vi "Module Interface.vi"(9 "rSubPanel":refnum<vi>, 10 "模块定义":T1={"模块名称"="系统", "项定义"=[{"项名"="设置", "符号图形路径"=path "D:/GitHub/UI-Frame/Pictures/Setting.png"}]}) -> ()   [LabVIEW 2020, in "Grouped Interface.lvlib"]
doc: "This template is based off of the Queued Message Handler design pattern and the Queued Message Handler project template that ships with LabVIEW.\n\nThe main difference is that the queue is private to this module and communication between modules is performed via Broadcast and Request events.\n\nRequest events are wrapped in public API methods and are handled in the Event Handling Loop (EHL) of this VI. Any module can register for Broadcast events sent by this module. The EHL generates messages based on user interface actions.\n\nThe Message Handling Loop (MHL) processes messages generated by the EHL, or by other messages. The messages are string values, so new messages can be added easily to the Message Cases case structure in the MHL. Each message cluster can also provide an optional value for Message Data, which is a variant that can be converted to whatever message-specific data is required.\n_____\nBased on DQMH Project Template 7.0.1.1316."
uses:
  Grouped Interface.lvlib
  <vilib>/Utility/miscctls.llb/LVRectTypeDef.ctl
  Module Definition--cluster.ctl
  Function Item--cluster.ctl
  <vilib>/Utility/miscctls.llb/LVPointTypeDef.ctl
  Window Size Change Arguments--cluster.ctl
  Item Selected Arguments--cluster.ctl
  50509386-df6b-4aff-9ba7-6a02358ed2a7.vi
  9a1344ca-f08d-4af5-a95b-0a8b33b9373c.vi
  7b477b35-5c05-4333-a059-2302209bca0e.vi
  3a33a204-8fa2-46f4-980e-14e97128f476.vi
  233c5268-b16d-435e-a8e5-754348a8c1c8.vi
  191d84f1-7d0a-4105-9754-8d98ffe8b58e.vi
  <userlib>/_NEVSTOP/Communicable State Machine(CSM)/AdvanceAPI/CSM - Revert Arguments-Safe String.vi
  <userlib>/_NEVSTOP/Communicable State Machine(CSM)/_Shared/Trim Single-line Text.vi
  <userlib>/_NEVSTOP/Communicable State Machine(CSM)/AdvanceAPI/CSM - Make String Arguments Safe.vi
  <userlib>/_NEVSTOP/Communicable State Machine(CSM)/AdvanceAPI/CSM - Break Down Multiple States String.vi
  <userlib>/_NEVSTOP/Communicable State Machine(CSM)/AdvanceAPI/CSM - Compact Multiple States.vi
  <userlib>/_NEVSTOP/Communicable State Machine(CSM)/AdvanceAPI/CSM - Keywords.vi
  <userlib>/_NEVSTOP/Communicable State Machine(CSM)/addons/API-String-Arugments-Support/_Support/Data To API String Arguments.vi
  <userlib>/_NEVSTOP/Communicable State Machine(CSM)/addons/API-String-Arugments-Support/_Support/Convert API String Arguments to Data(variant).vi
  <userlib>/_NEVSTOP/Communicable State Machine(CSM)/Communicable State Machine.lvlib
panel:
  out "窗口边界":T3
  in  "界面单元":T4={"ModuleName"="", "FunctionList"=0, "展收按钮"=TRUE, "Spacer"=""}
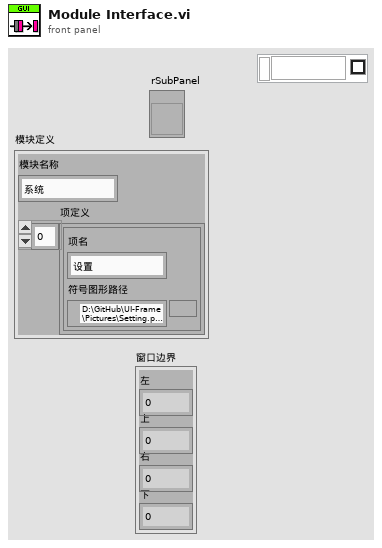
[diagram p1: front panel]
types:
  T1 = typedef "Grouped Interface.lvlib/Module Definition--cluster.ctl" = cluster{"模块名称":string, "项定义":T2[]}
  T2 = typedef "Grouped Interface.lvlib/Function Item--cluster.ctl" = cluster{"项名":string, "符号图形路径":path}
  T3 = typedef "LVRectTypeDef.ctl" = cluster{"Left":i16, "Top":i16, "Right":i16, "Bottom":i16}
  T4 = cluster{"ModuleName":string, "FunctionList":i32, "展收按钮":bool, "Spacer":string}
  T5 = enum32{"Invalid", "Standard", "Closed", "Hidden", "Minimized", "Maximized"}
  T6 = enum32{"invalid app kind", "Development System", "Run Time System", "Student Edition", "Embedded LabVIEW", "Evaluation", "Custom"}
  T7 = typedef "LVPointTypeDef.ctl" = cluster{"Horizontal":i16, "Vertical":i16}
  T8 = typedef "Grouped Interface.lvlib/Window Size Change Arguments--cluster.ctl" = cluster{"Module Name":string, "Window Size":T3}
  T9 = typedef "Grouped Interface.lvlib/Item Selected Arguments--cluster.ctl" = cluster{"Module Name":string, "Item Name":string}
  T10 = cluster{"Item Name":string, "New Item Name":string}
  T11 = typedef "Communicable State Machine.lvlib/_CSM_Response Source Message.ctl" = cluster{"‘State":string, "’Arguments":string, "’Error":errorcluster}
  T12 = cluster{"Current VI Reference":refnum<vi>, "Close Panel on Exit?":bool}
  T13 = cluster{"Core":cluster{"Current VI Reference":refnum<vi>, "Close Panel on Exit?":bool}, "界面单元":refnum<vi>, "ModuleName":refnum<vi>, "FunctionList":refnum<vi>, "Disabled Items":string[]}
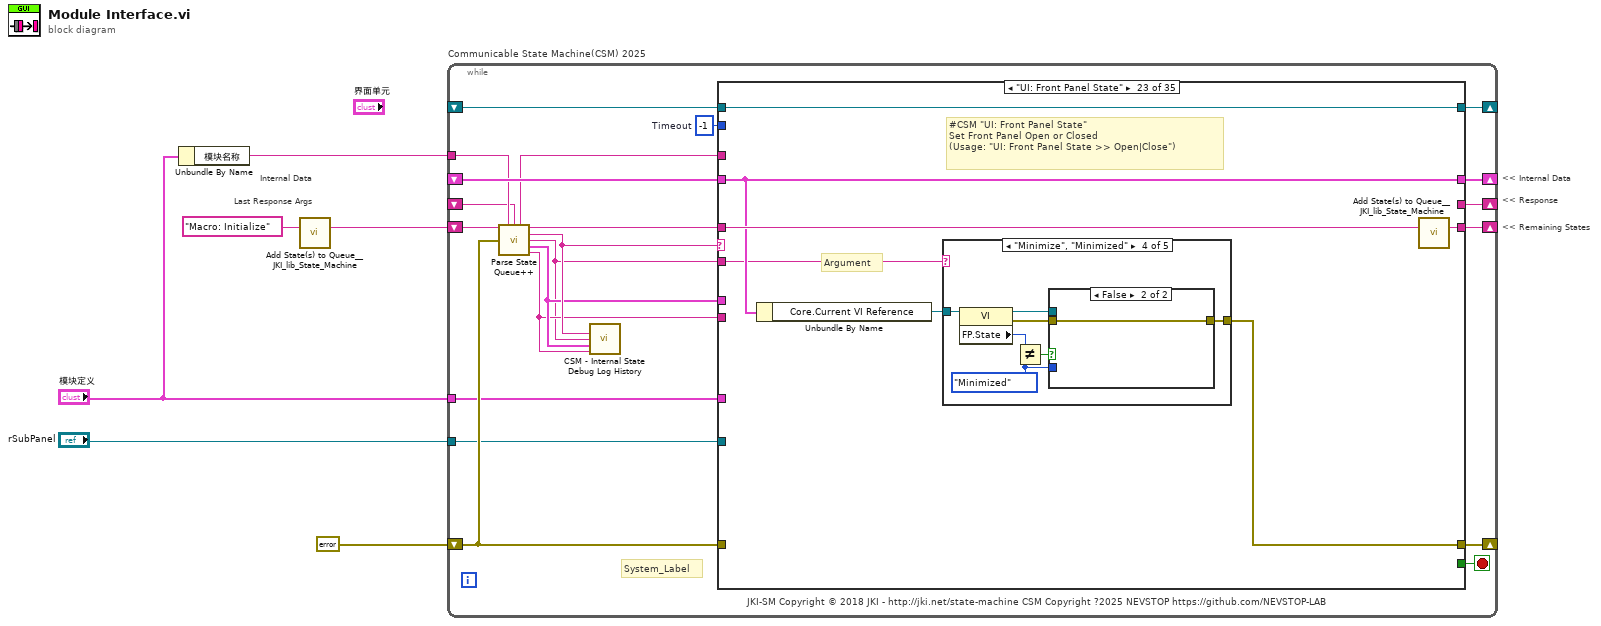
[diagram p0: block diagram]
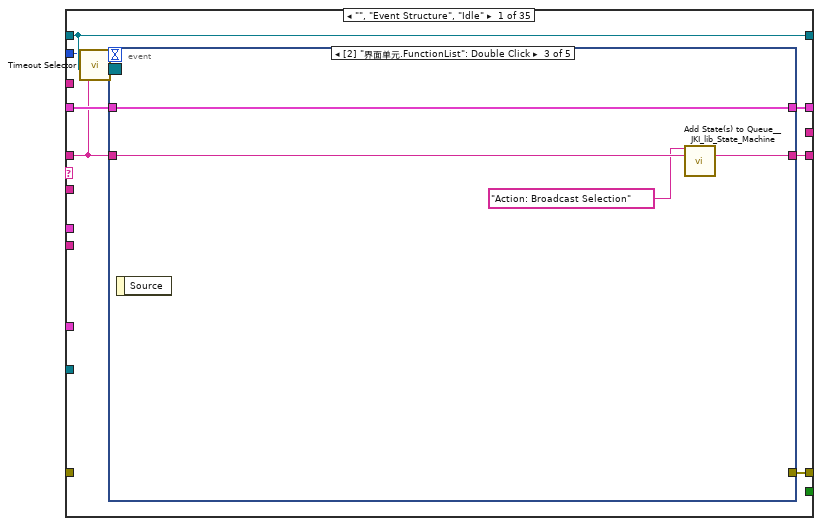
[diagram p2: hidden frame]
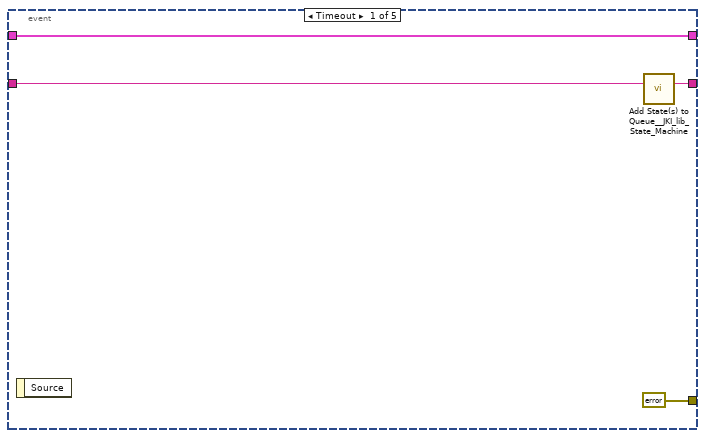
[diagram p3: hidden frame]
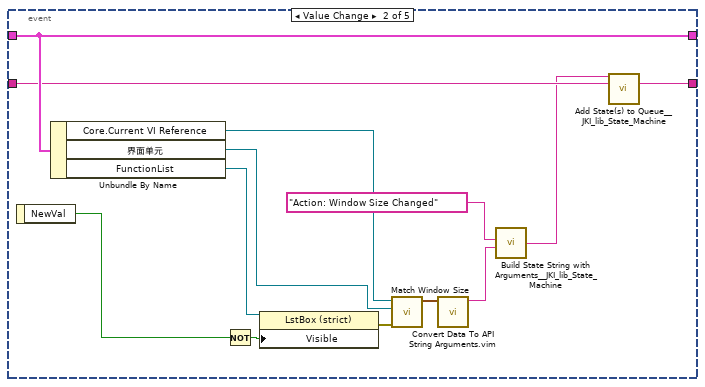
[diagram p4: hidden frame]
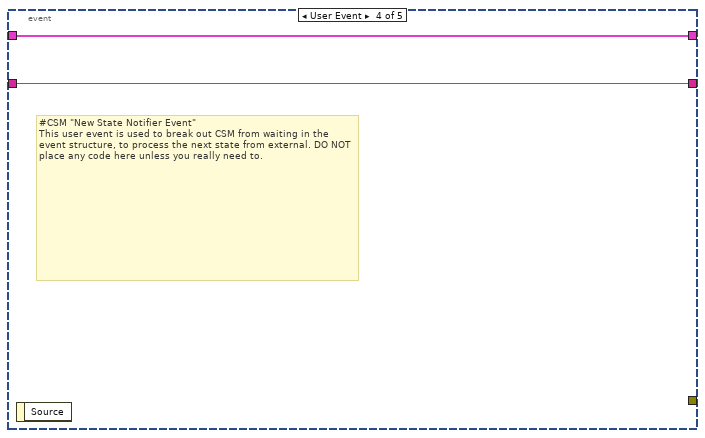
[diagram p5: hidden frame]
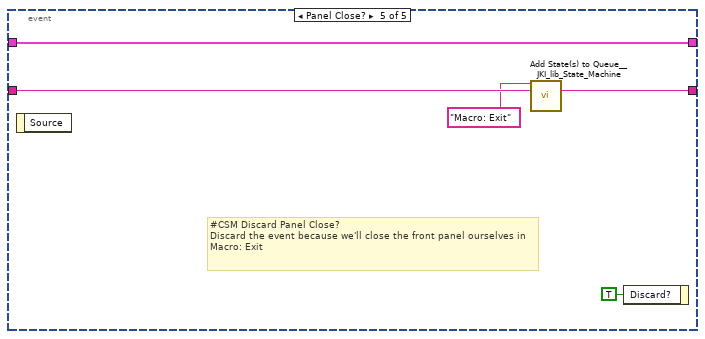
[diagram p6: hidden frame]
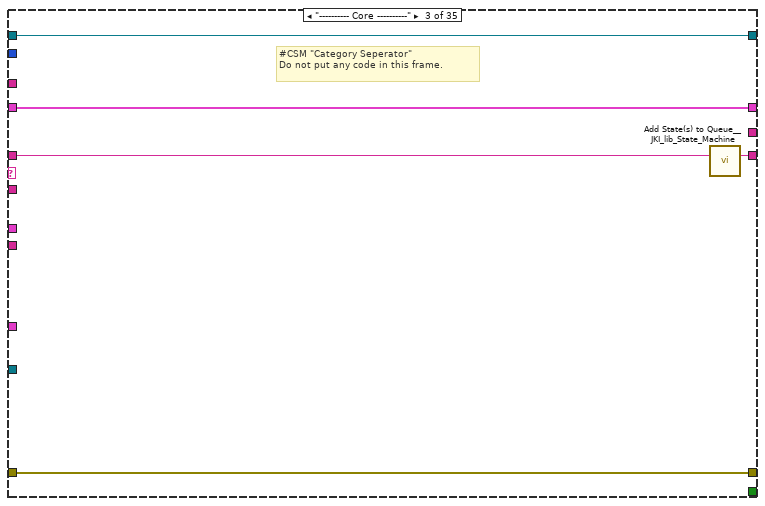
[diagram p8: hidden frame]
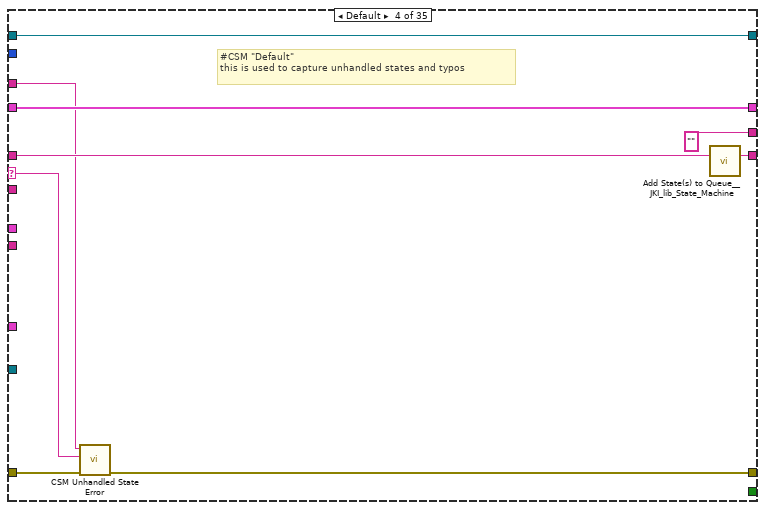
[diagram p9: hidden frame]
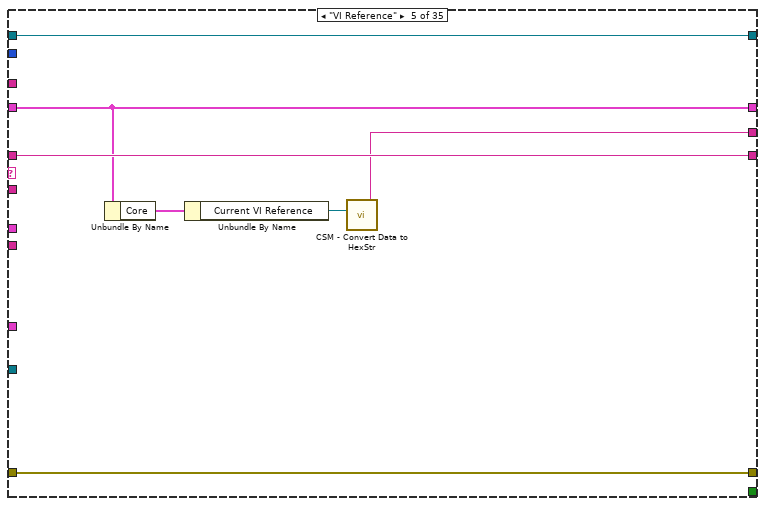
[diagram p10: hidden frame]
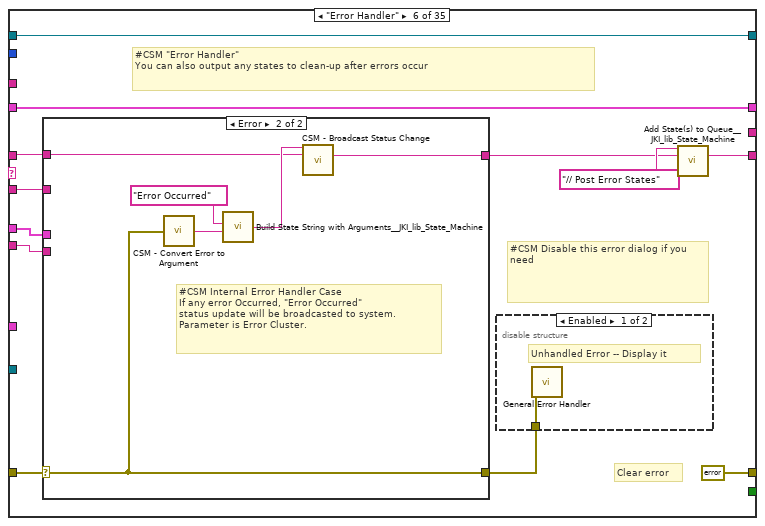
[diagram p11: hidden frame]
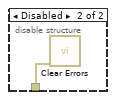
[diagram p12: hidden frame]
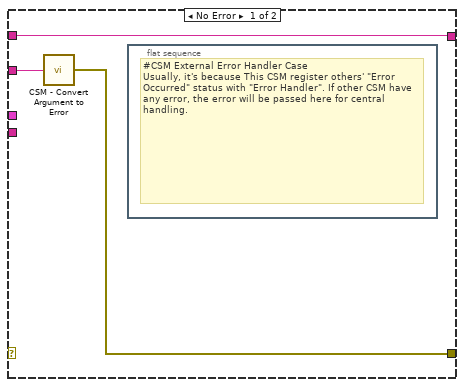
[diagram p13: hidden frame]
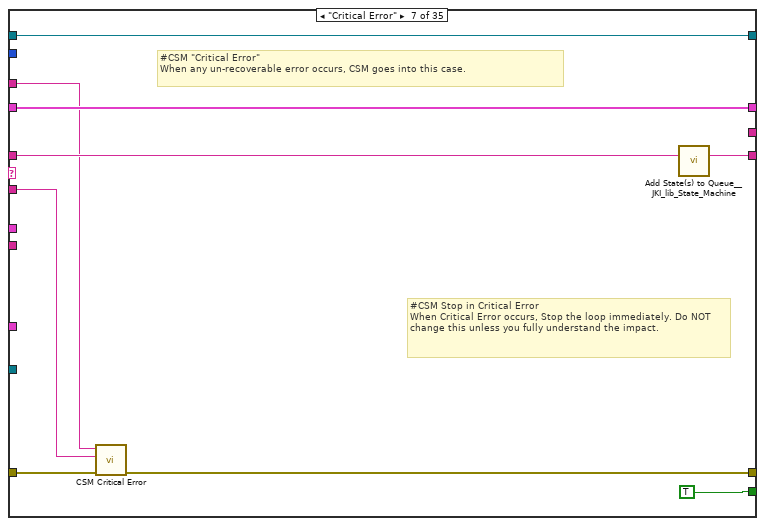
[diagram p14: hidden frame]
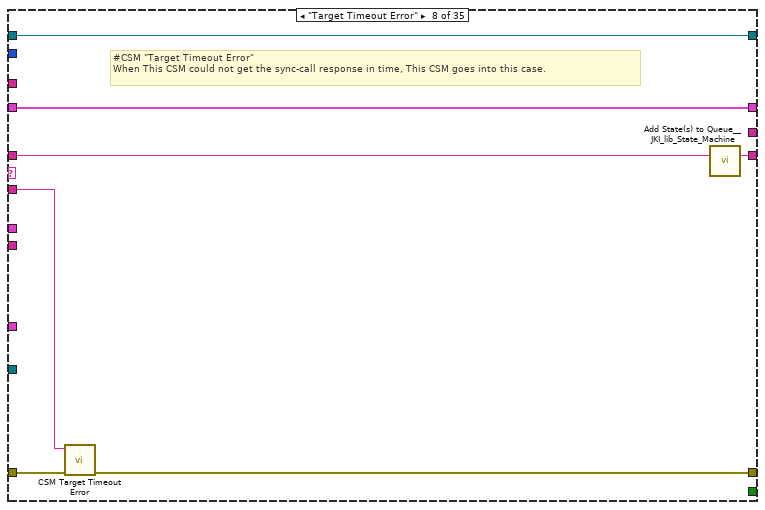
[diagram p15: hidden frame]
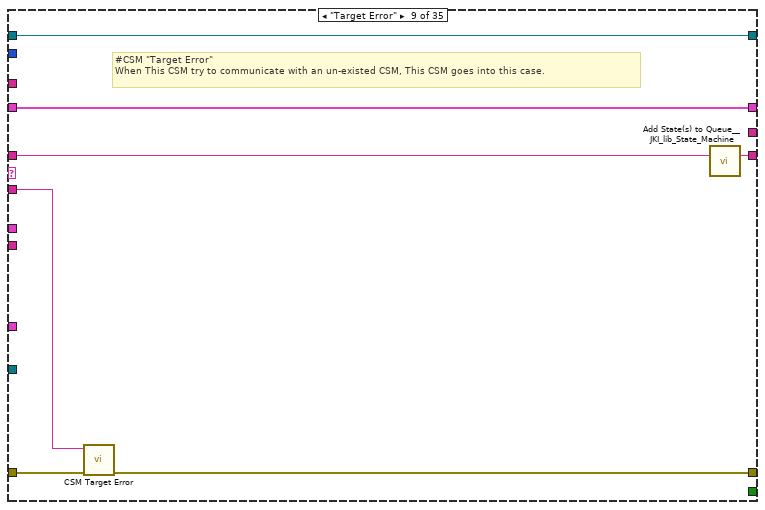
[diagram p16: hidden frame]
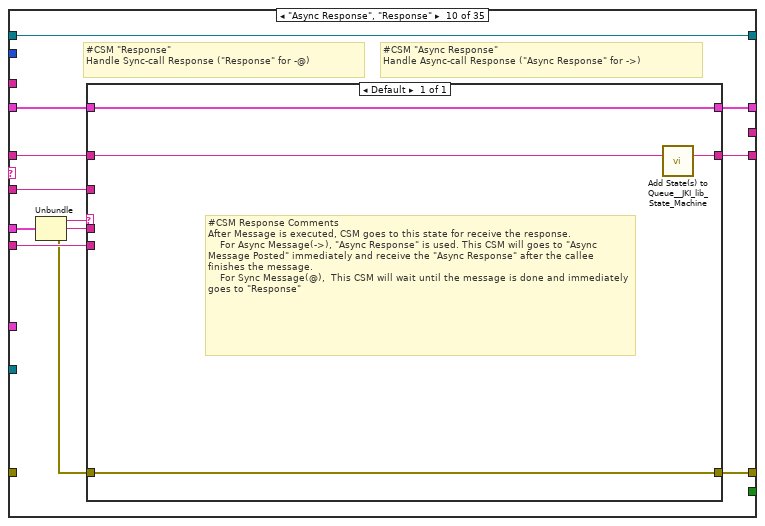
[diagram p17: hidden frame]
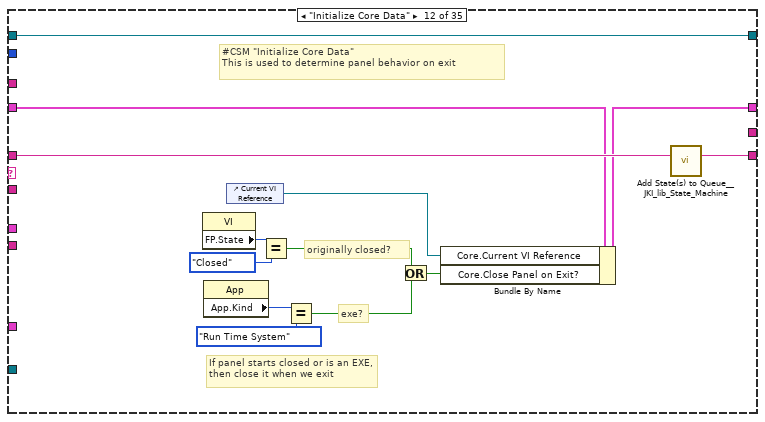
[diagram p19: hidden frame]
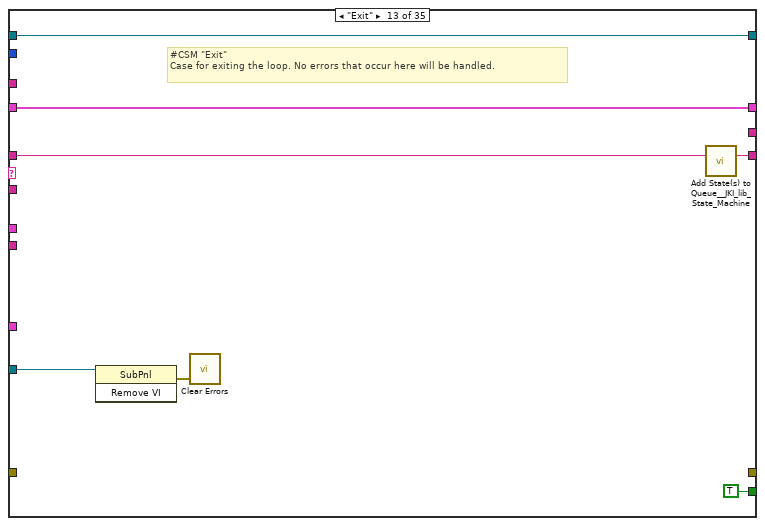
[diagram p20: hidden frame]
diagram:
  # "Last Response Args"
  # "Internal Data"
  # "<< Internal Data"
  # "<< Response"
  # "<< Remaining States"
  n1 = Unbundle By Name("模块定义") -> ("模块名称"=w3:string)
  n2 = call <vilib>:"Add State(s) to Queue__JKI_lib_State_Machine.vi"("State(s) in (\"\")"="Macro: Initialize" ("Init State(\"Macro: Initialize\")")) -> ("States Out"=w4:string)  [unwired: 14 in]
  n3 = while "Communicable State Machine(CSM) 2025" {
    shift-right: [w22] -> _
    shift-left: _ -> [w21]
    shift-right: [w25] -> _
    shift-left: errorcluster {"status"=FALSE, "code"=0, "source"=""} ("error out") -> [w19]
    shift-right: [w24] -> _
    shift-left: w4 -> [w26]
    tunnel: w3 -> [w15]
    shift-right: [w18] -> _
    shift-left: _ -> [w10]
    shift-right: [w17] -> _
    shift-left: _ -> [w16]
    tunnel: "模块定义" -> [w8]
    tunnel: "rSubPanel" -> [w7]
    stop <- w23 stop-if-true
    w20 = -1  # Timeout
    # "System_Label"
    # "JKI-SM Copyright © 2018 JKI - http://jki.net/state-machine CSM Copyright ?2025 NEVSTOP https://github.com/NEVSTOP-LAB"
    n4 = call <userlib>:"Parse State Queue++.vi"("State Queue"=w26, "Name (\"\" to Use UUID)"=w15, "Response Arguments"=w10, "Previous Error"=w19) -> ("Name Used"=w11:string, "Remaining States"=w27:string, "Current State"=w14:string, "Arguments"=w9:string, "Additional Information"=w13:T11, "Source CSM"=w12:string)  [unwired: 6 in]
    n5 = call <userlib>:"CSM - Internal State Debug Log History.vi"("State"=w14, "Arguments (\"\")"=w9, ">> Response Source Message >>"=w13, "Source (\"\")"=w12) -> ()  [unwired: 11 in, 1 out]
    n6 = case shown="\"UI: Front Panel State\"" w14 {
      selector: w14 -> [_ _ _ w74 _ _ _ _ _ _ _ _ _ _ _ _ _ _ _ _ _ _ _ _ _ _ _ _ _ _ _ _ _ _ _]
      tunnel: w27 -> [w28 w66 w71 w80 w86 w92 w118 w126 w133 w143 w152 w165 w172 w176 w185 w191 w195 w202 w206 w210 w230 w236 w247 w311 w316 w327 w330 w334 w337 w341 w352 w356 w389 w409 w432]
      tunnel: w9 -> [_ _ _ _ _ w90 w114 w121 w129 w137 _ _ _ _ _ _ _ _ _ _ _ w232 w242 _ _ _ _ _ _ _ w344 _ w379 w399 w426]
      tunnel: w21 -> [w34 w65 w68 w78 w85 w98 w119 w124 w131 w141 w151 w159 w170 w174 _ w187 w193 w201 w205 w208 w226 w234 w244 w309 w314 w325 w329 w333 w336 w339 w354 w359 w380 w398 w421]
      tunnel: [w33 _ w69 w72 w87 errorcluster {"status"=FALSE, "code"=0, "source"=""} ("error out") w111 w120 w127 w140 _ _ _ _ _ w188 _ w196 w204 _ _ w233 w245 _ _ _ _ _ _ _ _ _ _ _ _] -> w25
      tunnel: w19 -> [_ _ w69 w73 w87 w96 w112 w122 w128 _ _ _ _ _ _ _ _ _ _ _ _ _ _ _ _ _ _ _ _ _ _ _ _ _ _]
      tunnel: [w35 w66 w70 w79 w86 w94 w117 w125 w132 w144 w152 w164 w171 w175 w184 w190 w194 w202 w206 w209 w229 w235 w246 w310 w315 w326 w330 w334 w337 w340 w351 w357 w388 w408 w431] -> w24
      tunnel: [_ _ _ _ _ _ TRUE _ _ _ _ _ TRUE _ _ _ _ _ _ _ _ _ _ _ _ _ _ _ _ _ _ _ _ _ _] -> w23
      tunnel: [w32 w65 w68 w78 w85 w98 w119 w124 w131 w142 w151 w163 w170 w174 w183 w187 w193 w201 w205 w208 w226 w234 w244 w309 w314 w325 w329 w333 w336 w339 w354 w359 w377 w397 w421] -> w22
      tunnel: w20 -> [w30 _ _ _ _ _ _ _ _ _ _ _ _ _ _ _ _ _ _ _ _ _ _ _ _ _ _ _ _ _ _ _ _ _ _]
      tunnel: w12 -> [_ _ _ _ _ w89 _ _ _ w138 _ _ _ _ _ _ _ _ _ _ _ _ _ _ _ _ _ _ _ _ _ _ _ _ _]
      tunnel: w13 -> [_ _ _ _ _ w88 _ _ _ w139 _ _ _ _ _ _ _ _ _ _ _ _ _ _ _ _ _ _ _ _ _ _ _ _ _]
      tunnel: [_ _ _ "" w81 _ _ _ _ _ _ _ _ _ _ _ _ _ _ _ _ _ _ _ _ _ _ "API1 Response" _ _ _ _ _ _ _] -> w18
      tunnel: [w31 w64 w67 w76 w84 w97 w115 w123 w130 w145 w150 w153 w168 w173 w181 w186 w192 w200 w203 w207 w228 w231 w241 w308 w312 w318 w328 w332 w335 w338 w353 w366 w387 w407 w430] -> w17
      tunnel: w16 -> [w31 w64 w67 w76 w84 w97 w115 w123 w130 w145 w150 w153 w168 w173 w181 w186 w192 _ w203 w207 w228 w231 w241 w308 w312 w318 w328 w332 w335 w338 w353 w366 w387 w407 w430]
      tunnel: w11 -> [_ _ _ w75 _ _ w113 _ _ _ _ _ _ _ _ _ _ w199 _ _ _ _ _ _ _ _ _ _ _ _ w347 w355 _ _ _]
      tunnel: w8 -> [_ _ _ _ _ _ _ _ _ _ _ _ _ _ _ _ _ _ _ _ w227 _ _ _ _ _ _ _ _ _ _ _ _ _ _]
      tunnel: w7 -> [_ _ _ _ _ _ _ _ _ _ _ _ w166 _ _ _ _ _ _ _ w221 _ _ _ _ _ _ _ _ _ _ _ _ _ _]
      frame "", "Event Structure", "Idle" {
        n7 = call <userlib>:"Timeout Selector.vi"("Remaining States"=w28, "Timeout Expected"=w30) -> ("Timeout"=w29:i32)  [unwired: 5 in]
        n8 = event shown="[2] \"界面单元.FunctionList\": Double Click" {
          selector: w31 -> [_ _ _ _ _]
          dyn-events: _ -> [_ _ _ _ _]
          timeout: w29 -> [_ _ _ _ _]
          tunnel: w28 -> [w39 w41 w54 w57 w63]
          tunnel: [w38 w42 w55 w57 w62] -> w35
          tunnel: w34 -> [w37 w48 w56 w58 w61]
          tunnel: [errorcluster {"status"=FALSE, "code"=0, "source"=""} ("error out") _ _ _ _] -> w33
          tunnel: [w37 w48 w56 w58 w61] -> w32
          event Timeout {
            n9 = event-data() -> ()  [unwired: 1 in, 1 out]
            n10 = call <vilib>:"Add State(s) to Queue__JKI_lib_State_Machine.vi"("State(s) in (\"\")"=w39) -> ("States Out"=w38:string)  [unwired: 14 in]
          }
          event "界面单元.展收按钮": Value Change {
            n11 = event-data() -> ("NewVal"=w49:bool)  [unwired: 1 in]
            n12 = Unbundle By Name(w48) -> ("Core.Current VI Reference"=w45:refnum<vi>, "界面单元"=w46:refnum<vi>, "FunctionList"=w47:refnum<vi>)
            n13 = Not(x=w49) -> (.not. x?=w51:bool)
            n14 = property class="LstBox (strict)"(reference=w47, "Visible"=w51) -> (error out=w52:errorcluster)  [unwired: 1 in, 1 out]
            n15 = call "Match Window Size.vi"("错误输入（无错误）"=w52, "界面单元"=w46, "VI输入"=w45) -> ("窗口边界"=w50:T3)  [unwired: 7 in, 1 out]
            n16 = call "Convert Data To API String Arguments.vim"("Data"=w50) -> ("API String"=w43:string)  [unwired: 7 in, 1 out]
            n17 = call <vilib>:"Build State String with Arguments__JKI_lib_State_Machine.vi"("Arguments (\"\")"=w43, "State"="Action: Window Size Changed") -> ("State with Arguments"=w40:string)  [unwired: 4 in]
            n18 = call <vilib>:"Add State(s) to Queue__JKI_lib_State_Machine.vi"("State(s) in Front (\"\")"=w40, "State(s) in (\"\")"=w41) -> ("States Out"=w42:string)  [unwired: 13 in]
          }
          event "界面单元.FunctionList": Double Click {
            n19 = event-data() -> ()  [unwired: 1 in, 1 out]
            n20 = call <vilib>:"Add State(s) to Queue__JKI_lib_State_Machine.vi"("State(s) in Front (\"\")"="Action: Broadcast Selection" ("State(s) in Front (\"\")"), "State(s) in (\"\")"=w54) -> ("States Out"=w55:string)  [unwired: 13 in]
          }
          event User Event {
            # "#CSM \"New State Notifier Event\"\nThis user event is used to break out CSM from waiting in the event structure, to process the next state from external. DO NOT place any code here unless you really need to."
            n21 = event-data() -> ()  [unwired: 1 in, 1 out]
          }
          event Panel Close? {
            # "#CSM Discard Panel Close?\nDiscard the event because we'll close the front panel ourselves in Macro: Exit"
            n22 = event-data() -> ()  [unwired: 1 in, 1 out]
            n23 = call <vilib>:"Add State(s) to Queue__JKI_lib_State_Machine.vi"("State(s) in Front (\"\")"="Macro: Exit", "State(s) in (\"\")"=w63) -> ("States Out"=w62:string)  [unwired: 13 in]
            n24 = event-data("Discard?"=TRUE) -> ()  [unwired: 1 in, 1 out]
          }
        }
      }
      frame "CSM Documentation" {
        # "#CSM State Syntax\n\n// Comment line, all text to the right of “//” will be ignored\n// Local Message Example\nDoSth: DoA >> Arguments\n\n// Sync Call Example\nAPI: xxxx >> Arguments -@ TargetModule\n\n// Async Call Example\nAPI: xxxx >> Arguments -> TargetModule\n\n// Async Call without Reply Example\nAPI: xxxx >> Arguments ->| TargetModule\n\n// Broadcast normal status:\nStatus >> StatusArguments  -><status>\n\n// Broadcast Interrupt status:\nInterrupt >> StatusArguments  -><interrupt>\n\n// Register Source Module's status to Handler Module\nStatus@Source Module >> Handler Module@Handler Module -><register>\n\n// Unegister Source Module's status\nStatus@Source Module >> Handler Module -><unregister>"
        # "#CSM README FIRST\n\nCommunicable State Machine(CSM) is a LabVIEW application framework that builds upon JKI State Machine(JKISM). It follows the pattern of JKISM and extends the keywords to describe message communication between modules, including concepts such as Sync-Message, Async-Message, Subscription/Unsubscription of status - essential elements for creating reusable code modules. For more information, please visit the CSM wiki: https://nevstop-lab.github.io/CSM-Wiki/\n\nFor instructions on JKI State Machine, visit: \n    http://jki.net/state-machine/\nFor information about CSM, visit: \n    https://github.com/NEVSTOP-LAB"
        # "#CSM \"Documentation\"\nCase for holding CSM Documenation"
      }
      frame "---------- Core ----------" {
        # "#CSM \"Category Seperator\"\nDo not put any code in this frame."
        n25 = call <vilib>:"Add State(s) to Queue__JKI_lib_State_Machine.vi"("State(s) in (\"\")"=w71) -> ("States Out"=w70:string)  [unwired: 14 in]
      }
      frame Default {
        # "#CSM \"Default\"\nthis is used to capture unhandled states and typos"
        n26 = call <userlib>:"CSM Unhandled State Error.vi"("error in (no error)"=w73, "Undefined State"=w74, "CSM Name"=w75) -> ("error out"=w72:errorcluster)  [unwired: 8 in]
        n27 = call <vilib>:"Add State(s) to Queue__JKI_lib_State_Machine.vi"("State(s) in (\"\")"=w80) -> ("States Out"=w79:string)  [unwired: 14 in]
      }
      frame "VI Reference" {
        n28 = Unbundle By Name(w85) -> ("Core"=w83:T12)
        n29 = Unbundle By Name(w83) -> ("Current VI Reference"=w82:refnum<vi>)
        n30 = call <userlib>:"CSM - Convert Data to HexStr.vi"("Variant"=w82) -> ("HEX String (0-9,A-F)"=w81:string)  [unwired: 8 in]
      }
      frame "Error Handler" {
        # "#CSM Disable this error dialog if you need"
        # "#CSM \"Error Handler\"\nYou can also output any states to clean-up after errors occur"
        # "Clear error"
        n31 = case shown="Error" w96 {
          selector: w96 -> [_ w105]
          tunnel: [w103 w107] -> w93
          tunnel: w92 -> [w103 w106]
          tunnel: [w102 w105] -> w91
          tunnel: w90 -> [w104 _]
          tunnel: w89 -> [_ _]
          tunnel: w88 -> [_ _]
          frame No Error {
            n32 = call <userlib>:"CSM - Convert Argument to Error.vi"("Argument"=w104) -> ("Error"=w102:errorcluster)  [unwired: 4 in]
            n33 = flat-sequence {
              frame #0 {
                # "#CSM External Error Handler Case\nUsually, it's because This CSM register others' \"Error Occurred\" status with \"Error Handler\". If other CSM have any error, the error will be passed here for central handling."
              }
            }
          }
          frame Error {
            # "#CSM Internal Error Handler Case \nIf any error Occurred, \"Error Occurred\" \nstatus update will be broadcasted to system.\nParameter is Error Cluster."
            n34 = call <userlib>:"CSM - Convert Error to Argument.vi"("Error"=w105) -> ("Argument"=w109:string)  [unwired: 4 in]
            n35 = call <vilib>:"Build State String with Arguments__JKI_lib_State_Machine.vi"("Arguments (\"\")"=w109, "State"="Error Occurred" ("Status with Arguments")) -> ("State with Arguments"=w108:string)  [unwired: 4 in]
            n36 = call <userlib>:"CSM - Broadcast Status Change.vi"("Status With Arguments"=w108, "State Queue"=w106) -> ("Remaining States"=w107:string)  [unwired: 13 in]
          }
        }
        n37 = disable-structure shown="Enabled" {
          disable-tunnel: w91 -> [w100 w101]
          frame Enabled {
            # "Unhandled Error -- Display it"
            n38 = call <vilib>:"General Error Handler.vi"("error in (no error)"=w100) -> ()  [unwired: 10 in, 5 out]
          }
          frame Disabled {
            n39 = call <vilib>:"Clear Errors.vi"("error in (no error)"=w101) -> ()  [unwired: 5 in, 2 out]
          }
        }
        n40 = call <vilib>:"Add State(s) to Queue__JKI_lib_State_Machine.vi"("State(s) in Front (\"\")"="// Post Error States", "State(s) in (\"\")"=w93) -> ("States Out"=w94:string)  [unwired: 13 in]
      }
      frame "Critical Error" {
        # "#CSM \"Critical Error\"\nWhen any un-recoverable error occurs, CSM goes into this case."
        # "#CSM Stop in Critical Error\nWhen Critical Error occurs, Stop the loop immediately. Do NOT change this unless you fully understand the impact."
        n41 = call <userlib>:"CSM Critical Error.vi"("error in (no error)"=w112, "Arugments (As Reason)"=w114, "CSM Name"=w113) -> ("error out"=w111:errorcluster)  [unwired: 8 in]
        n42 = call <vilib>:"Add State(s) to Queue__JKI_lib_State_Machine.vi"("State(s) in (\"\")"=w118) -> ("States Out"=w117:string)  [unwired: 14 in]
      }
      frame "Target Timeout Error" {
        # "#CSM \"Target Timeout Error\"\nWhen This CSM could not get the sync-call response in time, This CSM goes into this case."
        n43 = call <userlib>:"CSM Target Timeout Error.vi"("error in (no error)"=w122, "Arguments (As CSM Name)"=w121) -> ("error out"=w120:errorcluster)  [unwired: 9 in]
        n44 = call <vilib>:"Add State(s) to Queue__JKI_lib_State_Machine.vi"("State(s) in (\"\")"=w126) -> ("States Out"=w125:string)  [unwired: 14 in]
      }
      frame "Target Error" {
        # "#CSM \"Target Error\"\nWhen This CSM try to communicate with an un-existed CSM, This CSM goes into this case."
        n45 = call <userlib>:"CSM Target Error.vi"("error in (no error)"=w128, "Arguments (As CSM Name)"=w129) -> ("error out"=w127:errorcluster)  [unwired: 9 in]
        n46 = call <vilib>:"Add State(s) to Queue__JKI_lib_State_Machine.vi"("State(s) in (\"\")"=w133) -> ("States Out"=w132:string)  [unwired: 14 in]
      }
      frame "Async Response", "Response" {
        # "#CSM \"Async Response\"\nHandle Async-call Response (\"Async Response\" for ->)"
        # "#CSM \"Response\"\nHandle Sync-call Response (\"Response\" for -@)"
        n47 = Unbundle(w139) -> ("‘State"=w136:string, "’Arguments"=w135:string, "’Error"=w134:errorcluster)
        n48 = case shown="Default" w136 {
          tunnel: [w146] -> w144
          tunnel: w143 -> [w147]
          tunnel: [w149] -> w142
          tunnel: w141 -> [w149]
          tunnel: [w148] -> w140
          tunnel: w134 -> [w148]
          tunnel: w138 -> [_]
          tunnel: w137 -> [_]
          tunnel: w135 -> [_]
          frame Default {
            # "#CSM Response Comments\nAfter Message is executed, CSM goes to this state for receive the response.\n    For Async Message(->), \"Async Response\" is used. This CSM will goes to \"Async Message Posted\" immediately and receive the \"Async Response\" after the callee finishes the message.\n    For Sync Message(@),  This CSM will wait until the message is done and immediately goes to \"Response\""
            n49 = call <vilib>:"Add State(s) to Queue__JKI_lib_State_Machine.vi"("State(s) in (\"\")"=w147) -> ("States Out"=w146:string)  [unwired: 14 in]
          }
        }
      }
      frame "Async Message Posted" {
        # "#CSM \"Async Message Posted\"\nAfter Async Message is posted (-> or ->| ), CSM goes to this state for post-action.\nYou can use Argument - State to tell which Async Message is called."
      }
      frame "Initialize Core Data" {
        # "#CSM \"Initialize Core Data\"\nThis is used to determine panel behavior on exit"
        # "originally closed?"
        # "exe?"
        # "If panel starts closed or is an EXE, then close it when we exit"
        n50 = property class="VI"() -> ("FP.State"=w156:T5)  [unwired: 2 in, 2 out]
        n51 = property class="App"() -> ("App.Kind"=w162:T6)  [unwired: 2 in, 2 out]
        n52 = control-ref of="Current VI Reference"() -> (w157:refnum<vi>)
        n53 = Equal?(x=w156, y=T5."Closed" ("Front Panel Window:State")) -> (x = y?=w154:bool)
        n54 = Equal?(x=w162, y=T6."Run Time System" ("Application:Kind")) -> (x = y?=w160:bool)
        n55 = Or(x=w154, y=w160) -> (x .or. y?=w158:bool)
        n56 = Bundle By Name(cluster=w159, "Core.Current VI Reference"=w157, "Core.Close Panel on Exit?"=w158) -> (w163:T13)
        n57 = call <vilib>:"Add State(s) to Queue__JKI_lib_State_Machine.vi"("State(s) in (\"\")"=w165) -> ("States Out"=w164:string)  [unwired: 14 in]
      }
      frame "Exit" {
        # "#CSM \"Exit\"\nCase for exiting the loop. No errors that occur here will be handled."
        n58 = invoke class="SubPnl" method="Remove VI"(reference=w166) -> (error out=w167:errorcluster)  [unwired: 2 in, 2 out]
        n59 = call <vilib>:"Clear Errors.vi"("error in (no error)"=w167) -> ()  [unwired: 5 in, 2 out]
        n60 = call <vilib>:"Add State(s) to Queue__JKI_lib_State_Machine.vi"("State(s) in (\"\")"=w172) -> ("States Out"=w171:string)  [unwired: 14 in]
      }
      frame "---------- Data ----------" {
        # "#CSM \"Category Seperator\"\nDo not put any code in this frame."
        n61 = call <vilib>:"Add State(s) to Queue__JKI_lib_State_Machine.vi"("State(s) in (\"\")"=w176) -> ("States Out"=w175:string)  [unwired: 14 in]
      }
      frame "Data: Initialize" {
        w177 = string[] []  # Disabled Items
        w182 = T12 {"Current VI Reference"=refnum, "Close Panel on Exit?"=FALSE}  # Core
        # "#CSM  do not delete - used by framework"
        # "#CSM Data names and types of shift register data are defined by this bundle."
        # "#CSM \"Data: Initialize\"\nInitialize the shift-register data, here.\n(data names are defined by what you wire into the bundle function)"
        n62 = control-ref of="界面单元"() -> (w180:refnum<vi>)
        n63 = control-ref of="FunctionList"() -> (w178:refnum<vi>)
        n64 = control-ref of="ModuleName"() -> (w179:refnum<vi>)
        n65 = Bundle("Core"=w182, "界面单元"=w180, "ModuleName"=w179, "FunctionList"=w178, "Disabled Items"=w177) -> (w183:T13)  [unwired: 1 in]
        n66 = call <vilib>:"Add State(s) to Queue__JKI_lib_State_Machine.vi"("State(s) in (\"\")"=w185) -> ("States Out"=w184:string)  [unwired: 14 in]
      }
      frame "Data: Cleanup" {
        # "#CSM \"Data: Cleanup\"\nCleanup any data and references, here.\n(this is called automatically, by the Macro: Exit)"
        n67 = Unbundle By Name(w187) -> ("Core.Current VI Reference"=w189:refnum<vi>)
        n68 = Close Reference(reference=w189) -> (error out=w188:errorcluster)  [unwired: 1 in]
        n69 = call <vilib>:"Add State(s) to Queue__JKI_lib_State_Machine.vi"("State(s) in (\"\")"=w191) -> ("States Out"=w190:string)  [unwired: 14 in]
      }
      frame "---------- Events ----------" {
        # "#CSM \"Category Seperator\"\nDo not put any code in this frame."
        n70 = call <vilib>:"Add State(s) to Queue__JKI_lib_State_Machine.vi"("State(s) in (\"\")"=w195) -> ("States Out"=w194:string)  [unwired: 14 in]
      }
      frame "Events: Register" {
        # "#CSM \"Events: Register\"\nRegister user event. New Message Event is registered to break CSM waiting in event structure by default."
        # "#CSM Register New Message Event\nRegister message event to break Waiting in Event structure."
        n71 = call <userlib>:"CSM - Get New State Notifier Event.vi"("Name (\"\" to Use UUID)"=w199) -> ("error out"=w197:errorcluster, "New State Notifier Event"=w198:refnum<user-event>)  [unwired: 9 in]
        n72 = register-events(error in=w197, w198) -> (reference out=w200:refnum<event-registration>, error out=w196:errorcluster)  [unwired: 1 in]
      }
      frame "Events: Unregister" {
        # "#CSM \"Events: Unregister\"\nUnregister user event."
        n73 = Unregister For Events(event registration refnum=w203) -> (error out=w204:errorcluster)  [unwired: 1 in]
      }
      frame "---------- UI ----------" {
        # "#CSM \"Category Seperator\"\nDo not put any code in this frame."
        n74 = call <vilib>:"Add State(s) to Queue__JKI_lib_State_Machine.vi"("State(s) in (\"\")"=w210) -> ("States Out"=w209:string)  [unwired: 14 in]
      }
      frame "UI: Initialize" {
        # "#CSM \"UI: Initialize\"\nInitialize the User Interface, here.\n(this is called automatically, by the Macro: Init)"
        n75 = control-ref of="FunctionList"() -> (w218:refnum<vi>)
        n76 = Unbundle By Name(w226) -> ("Core.Current VI Reference"=w220:refnum<vi>, "界面单元"=w222:refnum<vi>, "FunctionList"=w225:refnum<vi>, "ModuleName"=w224:refnum<vi>)
        n77 = property class="LstBox (strict)"(reference=w218, "Visible"=FALSE ("可见")) -> (error out=w216:errorcluster)  [unwired: 1 in, 1 out]
        n78 = property on="Pane" class="Pane"("Origin"=T7 {"Horizontal"=0, "Vertical"=0}) -> ()  [unwired: 2 in, 2 out]
        n79 = call "Initialize Function List.vi"("错误输入（无错误）"=w216, "模块定义"=w227, "rModuleName"=w224, "rFunctionList"=w225) -> ("错误输出"=w223:errorcluster)  [unwired: 7 in]
        n80 = call "Insert SubPanel.vi"("VI Ref"=w220, "Subpanel Ref"=w221) -> ("error out"=w215:errorcluster)  [unwired: 9 in]
        n81 = call "Match Window Size.vi"("错误输入（无错误）"=w223, "界面单元"=w222, "VI输入"=w220) -> ("窗口边界"=w214:T3)  [unwired: 7 in, 1 out]
        "窗口边界" <- w214
        n82 = call <vilib>:"Clear Errors.vi"("error in (no error)"=w215) -> ()  [unwired: 5 in, 2 out]
        n83 = call "Convert Data To API String Arguments.vim"("Data"=w214) -> ("API String"=w213:string)  [unwired: 7 in, 1 out]
        n84 = call <vilib>:"Build State String with Arguments__JKI_lib_State_Machine.vi"("Arguments (\"\")"=w213, "State"="Action: Window Size Changed") -> ("State with Arguments"=w212:string)  [unwired: 4 in]
        n85 = call <vilib>:"Add State(s) to Queue__JKI_lib_State_Machine.vi"("State(s) in Front (\"\")"=w212, "State(s) in (\"\")"=w230) -> ("States Out"=w229:string)  [unwired: 13 in]
      }
      frame "UI: Cursor Set" {
        # "Argument"
        # "#CSM \"UI: Cursor Set\"\nSet and Unset Cursor Busy.\n(Usage: \"UI: Cursor Set >> Busy|Idle\")"
        n86 = disable-structure shown="TARGET_TYPE!=Windows" {
          disable-tunnel: [w238 _] -> w233
          disable-tunnel: w232 -> [w237 _]
          frame condition #0 (active) {
            n87 = case shown="\"Idle\", Default" w237 {
              tunnel: [w239 w240] -> w238
              frame "Idle", Default {
                n88 = call <vilib>:"Unset Busy.vi"() -> ("error out"=w239:errorcluster)  [unwired: 11 in]
              }
              frame "Busy" {
                n89 = call <vilib>:"Set Busy.vi"() -> ("error out"=w240:errorcluster)  [unwired: 10 in, 1 out]
              }
            }
          }
          frame condition #1 {
          }
        }
        n90 = call <vilib>:"Add State(s) to Queue__JKI_lib_State_Machine.vi"("State(s) in (\"\")"=w236) -> ("States Out"=w235:string)  [unwired: 14 in]
      }
      frame "UI: Front Panel State" {
        # "Argument"
        # "#CSM \"UI: Front Panel State\"\nSet Front Panel Open or Closed\n(Usage: \"UI: Front Panel State >> Open|Close\")"
        n91 = Unbundle By Name(w244) -> ("Core.Current VI Reference"=w243:refnum<vi>)
        n92 = case shown="\"Minimize\", \"Minimized\"" w242 {
          tunnel: [w254 w267 w278 w290 w302] -> w245
          tunnel: w243 -> [w253 w265 w277 w289 w301]
          frame "Open", "Standard", Default {
            w248 = T5."Standard" ("State")
            n93 = property class="VI"(reference=w253) -> (reference out=w251:refnum<vi>, error out=w252:errorcluster, "FP.State"=w250:T5)  [unwired: 1 in]
            n94 = Not Equal?(x=w250, y=w248) -> (x != y?=w249:bool)
            n95 = case shown="True" w249 {
              tunnel: [w258 w260] -> w254
              tunnel: w252 -> [w257 w260]
              tunnel: w251 -> [w256 _]
              tunnel: w248 -> [w255 _]
              frame True {
                n96 = invoke class="VI" method="FP.Open"(reference=w256, error in=w257, "Activate"=TRUE, "State"=w255) -> (error out=w258:errorcluster)  [unwired: 1 in, 4 out]
              }
              frame False {
              }
            }
          }
          frame "Close", "Closed" {
            n97 = property class="VI"(reference=w265) -> (reference out=w264:refnum<vi>, error out=w266:errorcluster, "FP.State"=w262:T5)  [unwired: 1 in]
            n98 = Not Equal?(x=w262, y=T5."Closed" ("Front Panel Window:State")) -> (x != y?=w261:bool)
            n99 = case shown="True" w261 {
              tunnel: [w268 w271] -> w267
              tunnel: w266 -> [w268 w270]
              tunnel: w264 -> [_ w269]
              frame False {
              }
              frame True {
                n100 = invoke class="VI" method="FP.Close"(reference=w269, error in=w270) -> (error out=w271:errorcluster)  [unwired: 1 in, 2 out]
              }
            }
          }
          frame "Hidden", "Hide" {
            w272 = T5."Hidden" ("State")
            n101 = property class="VI"(reference=w277) -> (reference out=w275:refnum<vi>, error out=w276:errorcluster, "FP.State"=w274:T5)  [unwired: 1 in]
            n102 = Not Equal?(x=w274, y=w272) -> (x != y?=w273:bool)
            n103 = case shown="True" w273 {
              tunnel: [w282 w283] -> w278
              tunnel: w276 -> [w281 w283]
              tunnel: w275 -> [w280 _]
              tunnel: w272 -> [w279 _]
              frame True {
                n104 = invoke class="VI" method="FP.Open"(reference=w280, error in=w281, "State"=w279) -> (error out=w282:errorcluster)  [unwired: 2 in, 4 out]
              }
              frame False {
              }
            }
          }
          frame "Minimize", "Minimized" {
            w284 = T5."Minimized" ("State")
            n105 = property class="VI"(reference=w289) -> (reference out=w287:refnum<vi>, error out=w288:errorcluster, "FP.State"=w286:T5)  [unwired: 1 in]
            n106 = Not Equal?(x=w286, y=w284) -> (x != y?=w285:bool)
            n107 = case shown="False" w285 {
              tunnel: [w294 w295] -> w290
              tunnel: w288 -> [w293 w295]
              tunnel: w287 -> [w292 _]
              tunnel: w284 -> [w291 _]
              frame True {
                n108 = invoke class="VI" method="FP.Open"(reference=w292, error in=w293, "State"=w291) -> (error out=w294:errorcluster)  [unwired: 2 in, 4 out]
              }
              frame False {
              }
            }
          }
          frame "Maximize", "Maximized" {
            w296 = T5."Maximized" ("State")
            n109 = property class="VI"(reference=w301) -> (reference out=w299:refnum<vi>, error out=w300:errorcluster, "FP.State"=w298:T5)  [unwired: 1 in]
            n110 = Not Equal?(x=w298, y=w296) -> (x != y?=w297:bool)
            n111 = case shown="True" w297 {
              tunnel: [w306 w307] -> w302
              tunnel: w300 -> [w305 w307]
              tunnel: w299 -> [w304 _]
              tunnel: w296 -> [w303 _]
              frame True {
                n112 = invoke class="VI" method="FP.Open"(reference=w304, error in=w305, "State"=w303) -> (error out=w306:errorcluster)  [unwired: 2 in, 4 out]
              }
              frame False {
              }
            }
          }
        }
        n113 = call <vilib>:"Add State(s) to Queue__JKI_lib_State_Machine.vi"("State(s) in (\"\")"=w247) -> ("States Out"=w246:string)  [unwired: 14 in]
      }
      frame "---------- Macro ----------" {
        # "#CSM \"Category Seperator\"\nDo not put any code in this frame."
        n114 = call <vilib>:"Add State(s) to Queue__JKI_lib_State_Machine.vi"("State(s) in (\"\")"=w311) -> ("States Out"=w310:string)  [unwired: 14 in]
      }
      frame "Macro: Initialize" {
        w313 = "Data: Initialize\nInitialize Core Data\nEvents: Register\nUI: Initialize\nUI: Front Panel State >> Open"  # Data: Initialize Initialize Core Data Events: Register UI: Initialize UI: Front Panel State >> Open
        # "#CSM \"Macro: Initialize\"\nInitialization Macro (This is called once, when the VI starts)"
        n115 = call <vilib>:"Add State(s) to Queue__JKI_lib_State_Machine.vi"("State(s) in Front (\"\")"=w313, "State(s) in (\"\")"=w316) -> ("States Out"=w315:string)  [unwired: 13 in]
      }
      frame "Macro: Exit" {
        # "#CSM \"Macro: Exit\"\nExit Macro (This is called once, when the VI exits)"
        n116 = Unbundle By Name(w325) -> ("Core.Close Panel on Exit?"=w324:bool)
        n117 = Select(t="UI: Front Panel State >> Close", s=w324, f="") -> (s? t:f=w321:string)
        n118 = call <vilib>:"Add State(s) to Queue__JKI_lib_State_Machine.vi"("State(s) in Front (\"\")"="//Exit Sub-Modules ", "State(s) in (\"\")"=w321, "State(s) at Back (\"\")"="Data: Cleanup\nEvents: Unregister\nExit") -> ("States Out"=w319:string)  [unwired: 12 in]
        n119 = call <vilib>:"Add State(s) to Queue__JKI_lib_State_Machine.vi"("State(s) in Front (\"\")"=w319, "State(s) in (\"\")"=w327) -> ("States Out"=w326:string)  [unwired: 13 in]
      }
      frame "---------- API ----------" {
        # "#CSM \"Category Seperator\"\nDo not put any code in this frame."
      }
      frame "API: API1" {
        # "#CSM >> Source CSM >>\nIf you need to tell who triggered this state , use this string. If it's this case itself, this string is \"\"."
        # "#CSM >> Arguments >>\nDeal with the parameter if any"
        # "#CSM Response\nConnect this to return the response of your API"
        # "#CSM API Example\nCopy/Rename this case for your own API"
      }
      frame "API: API2" {
        # "#CSM API Example\nCopy/Rename this case for your own API"
      }
      frame "---------- Action ----------" {
        # "#CSM \"Category Seperator\"\nDo not put any code in this frame."
        n120 = call <vilib>:"Add State(s) to Queue__JKI_lib_State_Machine.vi"("State(s) in (\"\")"=w341) -> ("States Out"=w340:string)  [unwired: 14 in]
      }
      frame "Action: Window Size Changed" {
        # "#CSM \"Internal State\"\nThis category is used for holding internal states"
        n121 = call "Convert API String Arguments to Data.vim"("Reference Type"=T3 {"Left"=0, "Top"=0, "Right"=0, "Bottom"=0} ("窗口边界"), "API String"=w344) -> ("Data"=w342:T3)  [unwired: 6 in, 1 out]
        n122 = Bundle By Name(cluster=T8 {"Module Name"="", "Window Size"={"Left"=0, "Top"=0, "Right"=0, "Bottom"=0}}, "Module Name"=w347, "Window Size"=w342) -> (w346:T8)
        n123 = call "Convert Data To API String Arguments.vim"("Data"=w346) -> ("API String"=w345:string)  [unwired: 7 in, 1 out]
        n124 = call <vilib>:"Build State String with Arguments__JKI_lib_State_Machine.vi"("Arguments (\"\")"=w345, "State"="Window Size Changed") -> ("State with Arguments"=w350:string)  [unwired: 4 in]
        n125 = call <userlib>:"CSM - Broadcast Status Change.vi"("Status With Arguments"=w350, "State Queue"=w352) -> ("Remaining States"=w351:string)  [unwired: 13 in]
      }
      frame "Action: Broadcast Selection" {
        n126 = Unbundle By Name(w359) -> ("FunctionList"=w358:refnum<vi>)
        n127 = property class="LstBox (strict)"(reference=w358) -> ("Item Names"=w361:string[], "FocusRow"=w360:i32)  [unwired: 1 in, 2 out]
        n128 = Unbundle By Name(w359) -> ("Disabled Items"=w362:string[])
        n129 = Index Array(array=w361, index=w360) -> (element=w363:string)
        n130 = Search 1D Array(1D array=w362, element=w363) -> (index of element=w364:i32)  [unwired: 1 in]
        n131 = Less Than 0?(x=w364) -> (x < 0?=w365:bool)
        n132 = case shown="True" w365 {
          tunnel: w363 -> [_ w371]
          tunnel: [w367 w375] -> w357
          tunnel: w356 -> [w367 w376]
          tunnel: w355 -> [_ w370]
          frame False {
          }
          frame True {
            n133 = Bundle By Name(cluster=T9 {"Module Name"="", "Item Name"=""}, "Module Name"=w370, "Item Name"=w371) -> (w369:T9)
            n134 = call "Convert Data To API String Arguments.vim"("Data"=w369) -> ("API String"=w368:string)  [unwired: 7 in, 1 out]
            n135 = call <vilib>:"Build State String with Arguments__JKI_lib_State_Machine.vi"("Arguments (\"\")"=w368, "State"="Item Selected") -> ("State with Arguments"=w373:string)  [unwired: 4 in]
            n136 = call <userlib>:"CSM - Broadcast Status Change.vi"("Status With Arguments"=w373, "State Queue"=w376) -> ("Remaining States"=w375:string)  [unwired: 13 in]
          }
        }
      }
      frame "Action: Disable Item" {
        # "#CSM \"Internal State\"\nThis category is used for holding internal states"
        n137 = Unbundle By Name(w380) -> ("FunctionList"=w378:refnum<vi>)
        n138 = property class="LstBox (strict)"(reference=w378) -> (reference out=w384:refnum<vi>, "Item Names"=w381:string[])  [unwired: 1 in, 1 out]
        n139 = Unbundle By Name(w380) -> ("Disabled Items"=w386:string[])
        n140 = Search 1D Array(1D array=w381, element=w379) -> (index of element=w383:i32)  [unwired: 1 in]
        n141 = Greater Or Equal To 0?(x=w383) -> (x >= 0?=w382:bool)
        n142 = case shown="True" w382 {
          tunnel: w383 -> [_ w395]
          tunnel: w384 -> [_ w396]
          tunnel: w379 -> [_ w393]
          tunnel: [w390 w392] -> w385
          tunnel: w386 -> [w390 w391]
          frame False {
          }
          frame True {
            n143 = property class="LstBox (strict)"(reference=w396, "Active Row"=w395, "CellFontColor"=u32 9868950 ("活动行:单元格字体:颜色")) -> ()  [unwired: 1 in, 2 out]
            n144 = Build Array (concatenate)(w391, w393) -> (w392:string[])
          }
        }
        n145 = Bundle By Name(cluster=w380, "Disabled Items"=w385) -> (w377:T13)
        n146 = call <vilib>:"Add State(s) to Queue__JKI_lib_State_Machine.vi"("State(s) in (\"\")"=w389) -> ("States Out"=w388:string)  [unwired: 14 in]
      }
      frame "Action: Enable Item" {
        # "#CSM \"Internal State\"\nThis category is used for holding internal states"
        n147 = Unbundle By Name(w398) -> ("FunctionList"=w400:refnum<vi>)
        n148 = property class="LstBox (strict)"(reference=w400) -> (reference out=w404:refnum<vi>, "Item Names"=w401:string[])  [unwired: 1 in, 1 out]
        n149 = Unbundle By Name(w398) -> ("Disabled Items"=w405:string[])
        n150 = Search 1D Array(1D array=w401, element=w399) -> (index of element=w403:i32)  [unwired: 1 in]
        n151 = Greater Or Equal To 0?(x=w403) -> (x >= 0?=w402:bool)
        n152 = case shown="True" w402 {
          tunnel: w403 -> [_ w415]
          tunnel: w404 -> [_ w416]
          tunnel: w405 -> [w410 w413]
          tunnel: w399 -> [_ w412]
          tunnel: [w410 w411] -> w406
          frame False {
          }
          frame True {
            n153 = property class="LstBox (strict)"(reference=w416, "Active Row"=w415, "CellFontColor"=u32 7 ("活动行:单元格字体:颜色")) -> ()  [unwired: 1 in, 2 out]
            n154 = for {
              tunnel: w413 -> [w418] mode=indexing
              tunnel: w412 -> [w419]
              tunnel: [w418] -> w411 mode=indexing if=w417
              n155 = Not Equal?(x=w418, y=w419) -> (x != y?=w417:bool)
            }
          }
        }
        n156 = Bundle By Name(cluster=w398, "Disabled Items"=w406) -> (w397:T13)
        n157 = call <vilib>:"Add State(s) to Queue__JKI_lib_State_Machine.vi"("State(s) in (\"\")"=w409) -> ("States Out"=w408:string)  [unwired: 14 in]
      }
      frame "Action: Rename Item" {
        # "#CSM \"Category Seperator\"\nDo not put any code in this frame."
        n158 = Unbundle By Name(w421) -> ("FunctionList"=w420:refnum<vi>)
        n159 = call "Convert API String Arguments to Data.vim"("Reference Type"=T10 {"Item Name"="", "New Item Name"=""}, "API String"=w426) -> ("Data"=w425:T10)  [unwired: 6 in, 1 out]
        n160 = property class="LstBox (strict)"(reference=w420) -> (reference out=w429:refnum<vi>, "Item Names"=w428:string[])  [unwired: 1 in, 1 out]
        n161 = Unbundle By Name(w425) -> ("Item Name"=w424:string, "New Item Name"=w423:string)
        n162 = Search 1D Array(1D array=w428, element=w424) -> (index of element=w427:i32)  [unwired: 1 in]
        n163 = case shown="0, Default" w427 {
          selector: w427 -> [w437 _]
          tunnel: w423 -> [w436 _]
          tunnel: w428 -> [w435 _]
          tunnel: w429 -> [w433 _]
          frame 0, Default {
            n164 = Replace Array Subset(array=w435, new element=w436, index=w437) -> (w434:string[])
            n165 = property class="LstBox (strict)"(reference=w433, "Item Names"=w434) -> ()  [unwired: 1 in, 2 out]
          }
          frame -1 {
          }
        }
        n166 = call <vilib>:"Add State(s) to Queue__JKI_lib_State_Machine.vi"("State(s) in (\"\")"=w432) -> ("States Out"=w431:string)  [unwired: 14 in]
      }
    }
  }
